vi "read.vi"(8 "error in (no error)":errorcluster, 11 "SimAnalogHardware in":refnum<class "AnalogSimHardware.lvclass">) -> (0 "error out":errorcluster, 2 "outputs":u16[][](array[numeric]), 3 "SimAnalogHardware out":refnum<class "AnalogSimHardware.lvclass">)   [LabVIEW 2017, in "AnalogSimHardware.lvclass"]
doc: "Read data from the instrument"
uses:
  AnalogSimHardware.lvclass
  support/my_global.vi
panel:
  # "2d array of u16"
  # "If the number is greater than 32767 that means\nthe actual value is negativ and it is complementary code.\nBy subtracting 65536 this number will be converted to signed\ninteger."
  # "https://knowledge.ni.com/KnowledgeArticleDetails?id=kA00Z0000019YLoSAM&l=de-DE"
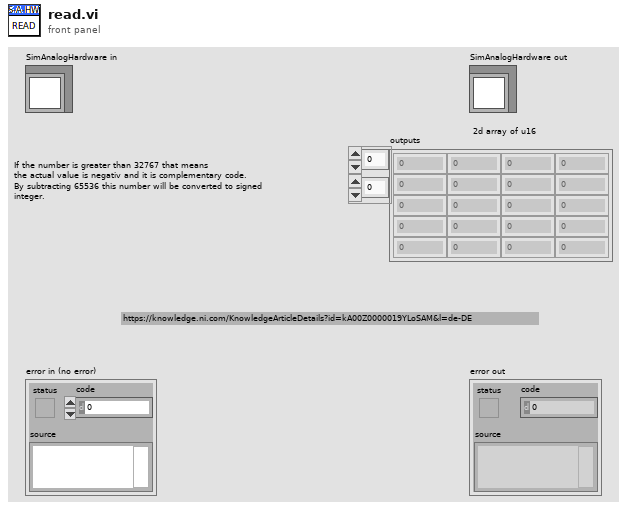
[diagram p1: front panel]
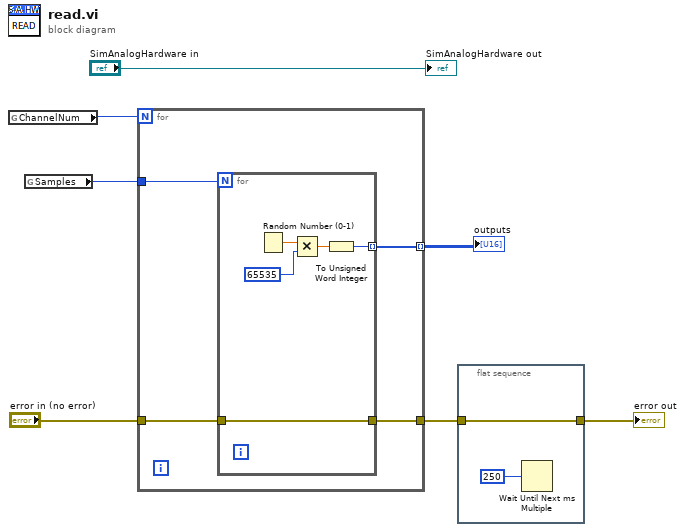
[diagram p0: block diagram]
diagram:
  n1 = global read "my_global.vi" "ChannelNum"() -> (w6:u32)
  n2 = global read "my_global.vi" "Samples"() -> (w5:u32)
  n3 = for {
    N: w6 -> [_]
    tunnel: w5 -> [w11]
    tunnel: [w10] -> w4 mode=indexing
    tunnel: "error in (no error)" -> [w9]
    tunnel: [w8] -> w2
    n4 = for {
      N: w11 -> [_]
      tunnel: [w13] -> w10 mode=indexing
      tunnel: w9 -> [w12]
      tunnel: [w12] -> w8
      n5 = Random Number (0-1)() -> (number: 0 to 1=w16:dbl)
      n6 = Multiply(x=w16, y=u16 65535) -> (x*y=w14:dbl)
      n7 = To Unsigned Word Integer(number=w14) -> (unsigned 16bit integer=w13:u16)
    }
  }
  "outputs" <- w4
  n8 = flat-sequence {
    tunnel: w2 -> [w17]
    tunnel: [w17] -> w1
    frame #0 {
      n9 = Wait Until Next ms Multiple(millisecond multiple=u32 250) -> ()  [unwired: 1 out]
    }
  }
  "error out" <- w1
  "SimAnalogHardware out" <- "SimAnalogHardware in"
